vi "cmdCode2Text.vi"(1 "CommandCode":string) -> (0 "CommandText":string)   [LabVIEW 2010]
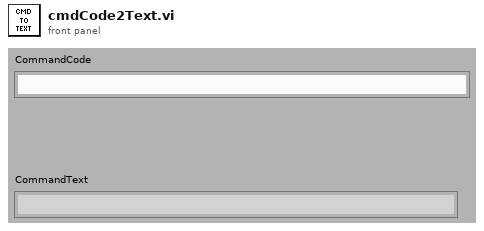
[diagram p1: front panel]
types:
  T1 = cluster{"address":string, "controlCode":string, "dataLength":dbl, "dataSection":string, "checkCode":string}
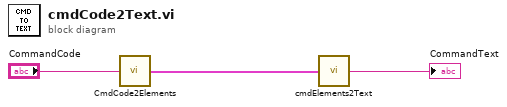
[diagram p0: block diagram]
diagram:
  n1 = call "CmdCode2Elements.vi"("CommandCode"="CommandCode") -> ("Elements"=w3:T1)
  n2 = call "cmdElements2Text.vi"("CodeElements"=w3) -> ("CommandText"=→"CommandText":string)
